vi "Berkeley Nucleonics 500 Series Initiate Pulses.vi"() -> ()   [LabVIEW 2013]
doc: "This VI is an example of how to use subVIs from the BNC 500 series driver to programmatically configure multiple channels and the system timer (To). This VI initializes the pulse generator, gets the number of channels in the unit, configures individual channel(s), configures the system timer (To), initiate pulse generation, and then closes communications with the pulse generator. By default the VI DOES NOT stop pulse generation when exiting!!! Not all trigger and gate features are supported by all models covered by this driver. Selection of an unsupported function will generate a software error and the command is not sent to the hardware.\n\n\nNotes:\n1) The pulse generator keypad is returned to \"Local\" mode when this VI terminates in order to restore manual control to the user.\n2) VISA Version 3.3 or higher must be installed to use this instrument driver."
uses:
  <instrlib>/Berkeley Nucleonics 500 Series/Examples/Support/Channel Parameters.ctl
  <instrlib>/Berkeley Nucleonics 500 Series/Examples/Support/System Parameters.ctl
  <instrlib>/Berkeley Nucleonics 500 Series/Berkeley Nucleonics 500 Series.lvlib
panel:
  out "System Parameters":T1={"Sys Period"=0.1, "Sys Mode"=enum."Normal", "Sys Burst #"=10, "Sys DC On"=10, "Sys DC Off"=10, "Sys State"=TRUE, "Sys Gate"=TRUE, "Sys Trig Edge"=TRUE, "Sys Ext Mode"=enum."Disabled", "Sys Trig Lev"=2.5, "Sys Gate Lev "=2.5, "Sys Gate Mode"=enum."Disabled"} {"Sys Gate Lev" format="%.4p"; "Sys Trig Lev" format="%.4p"; "Sys Period" format="%.6p"}
  out "Channel Parameters 2":T2[](array[typedef]) {"Chan Sync Source" items=["System (To)", "Channel A", "Channel B", "Channel C", "Channel D", "Channel E", "Channel F", "Channel G", "Channel H"]; "Chan Width" format="%.3p"; "Chan Delay" format="%.3p"; "Chan Lev Adjust" format="%.3p"; "Channel" items=["Channel A"=1, "Channel B"=2, "Channel C"=3, "Channel D"=4, "Channel E"=5, "Channel F"=6, "Channel G"=7, "Channel H"=8]}
  in  "VISA resource":refnum<visa-resource-name>="GPIB0::7::INSTR"
  in  "System Paramaters":T1={"Sys Period"=0.1, "Sys Mode"=enum."Normal", "Sys Burst #"=0, "Sys DC On"=10, "Sys DC Off"=20, "Sys State"=TRUE, "Sys Gate"=TRUE, "Sys Trig Edge"=TRUE, "Sys Ext Mode"=enum."Disabled", "Sys Trig Lev"=2.5, "Sys Gate Lev "=2.5, "Sys Gate Mode"=enum."Disabled"} {"Sys Gate Lev" format="%.4p"; "Sys Trig Lev" format="%.4p"; "Sys Period" format="%.6p"}
  in  "Channel Parameters":T2[](array[typedef])=[{"Channel"=1, "Chan State"=TRUE, "Chan Sync Source"=0, "Chan Gate Logic"=enum."Disabled", "Chan Mode"=enum."Normal", "Chan Wait #"=10, "Chan Delay"=0.01, "Chan Width"=0.01, "Chan Burst #"=10, "Chan DC On"=10, "Chan DC Off"=10, "Chan Polarity"=FALSE, "Chan MUX Value"=-1, "Chan Level Out"=enum."Adjustable", "Chan Lev Adjust"=0.0, "Chan Gate Mode"=enum."Disabled"}, {"Channel"=2, "Chan State"=TRUE, "Chan Sync Source"=0, "Chan Gate Logic"=enum."Disabled", "Chan Mode"=enum."Normal", "Chan Wait #"=20, "Chan Delay"=0.02, "Chan Width"=0.02, "Chan Burst #"=20, "Chan DC On"=20, "Chan DC Off"=20, "Chan Polarity"=FALSE, "Chan MUX Value"=-1, "Chan Level Out"=enum."35 Volt", "Chan Lev Adjust"=0.0, "Chan Gate Mode"=enum."Disabled"}, {"Channel"=3, "Chan State"=TRUE, "Chan Sync Source"=0, "Chan Gate Logic"=enum."Disabled", "Chan Mode"=enum."Normal", "Chan Wait #"=30, "Chan Delay"=0.03, "Chan Width"=0.03, "Chan Burst #"=30, "Chan DC On"=30, "Chan DC Off"=30, "Chan Polarity"=FALSE, "Chan MUX Value"=-1, "Chan Level Out"=enum."35 Volt", "Chan Lev Adjust"=0.0, "Chan Gate Mode"=enum."Disabled"}, {"Channel"=4, "Chan State"=TRUE, "Chan Sync Source"=0, "Chan Gate Logic"=enum."Disabled", "Chan Mode"=enum."Normal", "Chan Wait #"=40, "Chan Delay"=0.04, "Chan Width"=0.04, "Chan Burst #"=40, "Chan DC On"=40, "Chan DC Off"=40, "Chan Polarity"=FALSE, "Chan MUX Value"=-1, "Chan Level Out"=enum."35 Volt", "Chan Lev Adjust"=0.0, "Chan Gate Mode"=enum."Disabled"}] {"Chan Sync Source" items=["System (To)", "Channel A", "Channel B", "Channel C", "Channel D", "Channel E", "Channel F", "Channel G", "Channel H"]; "Chan Width" format="%.3p"; "Chan Delay" format="%.3p"; "Chan Lev Adjust" format="%.3p"; "Channel" items=["Channel A"=1, "Channel B"=2, "Channel C"=3, "Channel D"=4, "Channel E"=5, "Channel F"=6, "Channel G"=7, "Channel H"=8]}
  # "500 Series\nPulse Generator\nExample Program"
  # "Notes:\n1.  The channel parameters \"Burst #\", \"DC On\", \"DC Off\", and \"Adjustable\" are only updated when operating in the corresponding mode.\n2.  The system parameters  \"Burst #\", \"DC On\", \"DC Off\", and \"Trig Level\"` are only updated when operating in the corresponding mode."
  # "Input"
  # "Triggered"
  # "Gated"
  # "Mode"
  # "Burst"
  # "Duty\nCycle"
  # "Input"
  # "Normal\nSingle\nBurst"
  # "Burst"
  # "Duty Cycle"
  # "Output"
  # "Input"
  # "Triggered"
  # "Gated"
  # "Mode"
  # "Burst"
  # "Duty\nCycle"
  # "Input"
  # "Normal\nSingle\nBurst"
  # "Burst"
  # "Duty Cycle"
  # "Output"
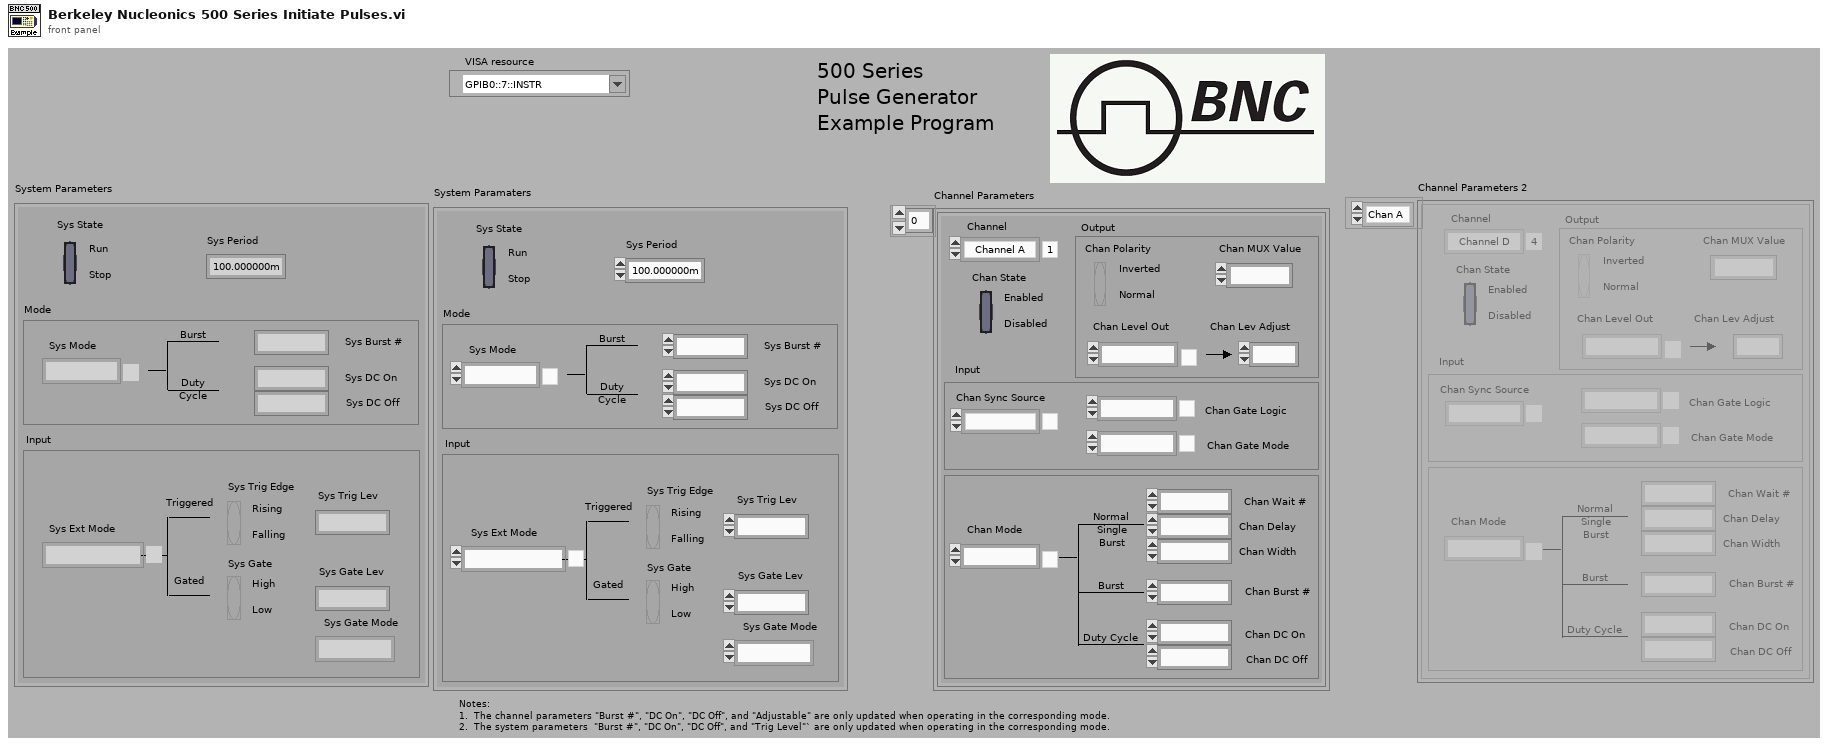
[diagram p1: front panel]
types:
  T1 = typedef "System Parameters.ctl" = cluster{"Sys Period":dbl, "Sys Mode":enum16{"Normal", "Single", "Burst", "Duty Cycle"}, "Sys Burst #":i32, "Sys DC On":i32, "Sys DC Off":i32, "Sys State":bool, "Sys Gate":bool, "Sys Trig Edge":bool, "Sys Ext Mode":enum16{"Disabled", "Triggered", "Gated", "Triggered & Gated"}, "Sys Trig Lev":dbl, "Sys Gate Lev ":dbl, "Sys Gate Mode":enum16{"Disabled", "Pulse Inhibit", "Output Inhibit", "Channel"}}
  T2 = typedef "Channel Parameters.ctl" = cluster{"Channel":i32, "Chan State":bool, "Chan Sync Source":i32, "Chan Gate Logic":enum16{"Disabled", "Low", "High"}, "Chan Mode":enum16{"Normal", "Single", "Burst", "Duty Cycle"}, "Chan Wait #":i32, "Chan Delay":dbl, "Chan Width":dbl, "Chan Burst #":i32, "Chan DC On":i32, "Chan DC Off":i32, "Chan Polarity":bool, "Chan MUX Value":i32, "Chan Level Out":enum16{"TTL", "Adjustable", "35 Volt", "Optical"}, "Chan Lev Adjust":dbl, "Chan Gate Mode":enum16{"Disabled", "Pulse Inhibit", "Output Inhibit"}}
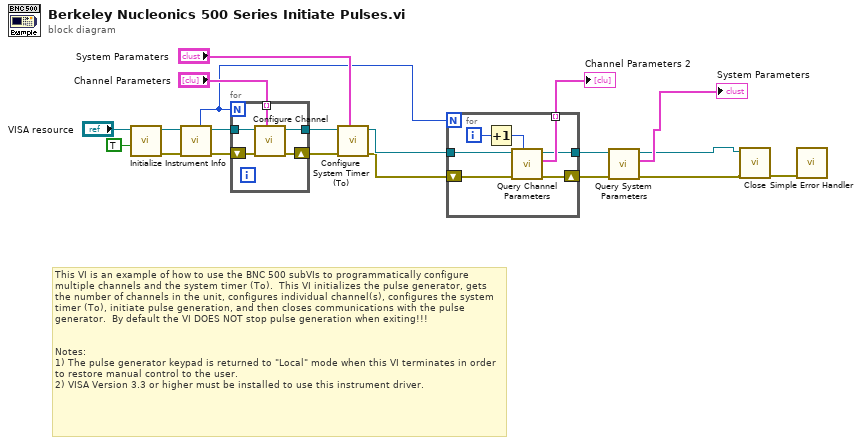
[diagram p0: block diagram]
diagram:
  # "This VI is an example of how to use the BNC 500 subVIs to programmatically configure multiple channels and the system timer (To).  This VI initializes the pulse generator, gets the number of channels in the unit, configures individual channel(s), configures the system timer (To), initiate pulse generation, and then closes communications with the pulse generator.  By default the VI DOES NOT stop pulse generation when exiting!!!\n\n\nNotes:\n1) The pulse generator keypad is returned to \"Local\" mode when this VI terminates in order to restore manual control to the user.\n2) VISA Version 3.3 or higher must be installed to use this instrument driver."
  n1 = call <instrlib>:"Initialize.vi"("Reset? (T: Yes)"=TRUE, "VISA resource name"="VISA resource") -> ("error out"=w14:errorcluster, "VISA resource name out"=w15:refnum<visa-resource-name>)  [unwired: 8 in]
  n2 = call <instrlib>:"Instrument Info.vi"("error in (no error)"=w14, "VISA resource name"=w15) -> ("error out"=w12:errorcluster, "VISA resource name out"=w16:refnum<visa-resource-name>, "Channels"=w1:i32)  [unwired: 6 in, 1 out]
  n3 = for {
    N: w1 -> [_]
    tunnel: [w25] -> w20
    tunnel: "Channel Parameters" -> [w24] mode=indexing
    tunnel: w16 -> [w23]
    shift-right: [w22] -> w13
    shift-left: w12 -> [w21]
    n4 = call <instrlib>:"Configure Channel.vi"("Chan Parameters"=w24, "error in (no error)"=w21, "VISA resource name"=w23) -> ("error out"=w22:errorcluster, "VISA resource name out"=w25:refnum<visa-resource-name>)  [unwired: 7 in]
  }
  n5 = call <instrlib>:"Configure System Timer (To).vi"("System Parameters"="System Paramaters", "error in (no error)"=w13, "VISA resource name"=w20) -> ("error out"=w4:errorcluster, "VISA resource name out"=w5:refnum<visa-resource-name>)  [unwired: 7 in]
  n6 = for {
    N: w1 -> [_]
    tunnel: w5 -> [w32]
    tunnel: [w31] -> w6 mode=indexing
    shift-right: [w29] -> w8
    shift-left: w4 -> [w30]
    tunnel: [w28] -> w9
    i -> [w27]
    n7 = Increment(x=w27) -> (x+1=w26:i32)
    n8 = call <instrlib>:"Query Channel Parameters.vi"("Channel (1:Chan A)"=w26, "error in (no error)"=w30, "VISA resource name"=w32) -> ("error out"=w29:errorcluster, "Chan Parameters"=w31:T2, "VISA resource name out"=w28:refnum<visa-resource-name>)  [unwired: 6 in]
  }
  "Channel Parameters 2" <- w6
  n9 = call <instrlib>:"Query System Parameters.vi"("error in (no error)"=w8, "VISA resource name"=w9) -> ("error out"=w2:errorcluster, "System Parameters"=→"System Parameters":T1, "VISA resource name out"=w3:refnum<visa-resource-name>)  [unwired: 7 in]
  n10 = call <instrlib>:"Close.vi"("error in (no error)"=w2, "VISA resource name"=w3) -> ("error out"=w11:errorcluster)  [unwired: 9 in]
  n11 = call <vilib>:"Simple Error Handler.vi"("error in (no error)"=w11) -> ()  [unwired: 4 in, 5 out]
